vi "NET_speech.vi"(8 "error in (no error)":errorcluster, 10 "Голос":i32=1, 11 "textToSpeak":string="А всем привет!") -> (0 "error out":errorcluster, 2 "Голоса":T1(array[cluster]))   [LabVIEW 2017]
uses:
  System.Speech
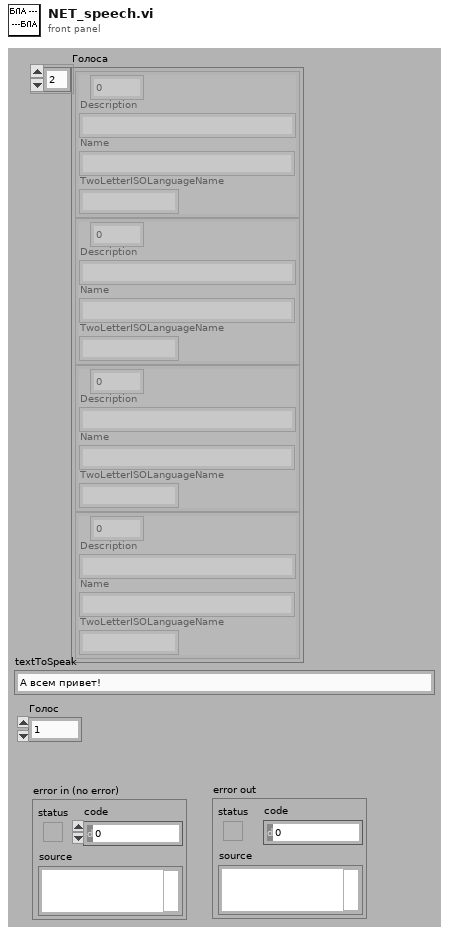
[diagram p1: front panel]
types:
  T1 = cluster{i32, "Description":string, "Name":string, "TwoLetterISOLanguageName":string}[]
  T2 = cluster{i32, "Description":string, "Name":string, "TwoLetterISOLanguageName":string}
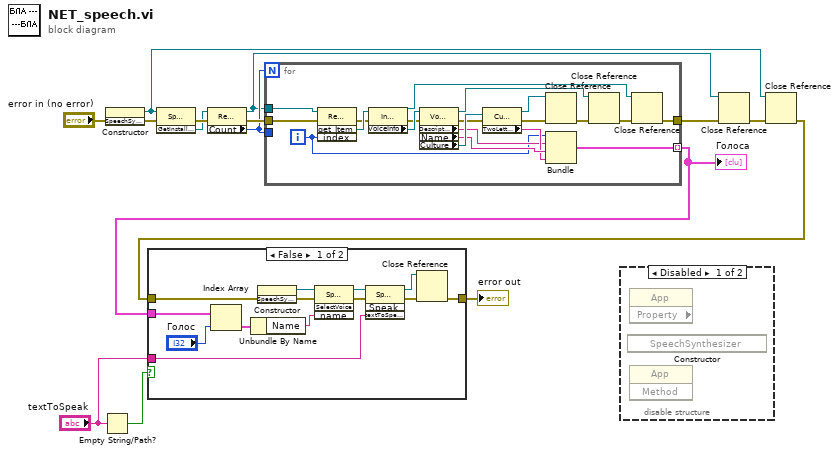
[diagram p0: block diagram]
diagram:
  n1 = Empty String/Path?(string/path="textToSpeak") -> (empty?=w5:bool)
  n2 = constructor class="SpeechSynthesizer"(error in="error in (no error)") -> (reference out=w7:refnum<k24>, error out=w15:errorcluster)  [unwired: 2 in, 1 out]
  n3 = invoke class="SpeechSynthesizer" method="GetInstalledVoices"(reference=w7, error in=w15) -> (error out=w14:errorcluster, "GetInstalledVoices"=w11:refnum<k24>)  [unwired: 1 in, 1 out]
  n4 = property class="ReadOnlyCollection`1[[System.Sp"(reference=w11, error in=w14) -> (reference out=w9:refnum<k24>, error out=w13:errorcluster, "Count"=w10:i32)
  n5 = for {
    N: w10 -> [_]
    tunnel: w9 -> [w35]
    tunnel: w10 -> [_]
    tunnel: [w28] -> w1 mode=indexing
    tunnel: w13 -> [w27]
    tunnel: [w17] -> w12
    i -> [w16]
    n6 = invoke class="ReadOnlyCollection`1[[System.Sp" method="get_Item"(reference=w35, error in=w27, "index"=w16) -> (error out=w26:errorcluster, "get_Item"=w34:refnum<k24>)  [unwired: 1 in, 2 out]
    n7 = property class="InstalledVoice"(reference=w34, error in=w26) -> (reference out=w18:refnum<k24>, error out=w25:errorcluster, "VoiceInfo"=w33:refnum<k24>)
    n8 = property class="VoiceInfo"(reference=w33, error in=w25) -> (reference out=w20:refnum<k24>, error out=w24:errorcluster, "Description"=w29:string, "Name"=w31:string, "Culture"=w32:refnum<k24>)
    n9 = property class="CultureInfo"(reference=w32, error in=w24) -> (reference out=w23:refnum<k24>, error out=w22:errorcluster, "TwoLetterISOLanguageName"=w30:string)
    n10 = Close Reference(reference=w23, error in (no error)=w22) -> (error out=w21:errorcluster)
    n11 = Bundle(w16, "Description"=w29, "Name"=w31, "TwoLetterISOLanguageName"=w30) -> (w28:T2)  [unwired: 1 out]
    n12 = Close Reference(reference=w20, error in (no error)=w21) -> (error out=w19:errorcluster)
    n13 = Close Reference(reference=w18, error in (no error)=w19) -> (error out=w17:errorcluster)
  }
  "Голоса" <- w1
  n14 = disable-structure shown="Disabled" {
    frame Disabled {
      n15 = constructor class="SpeechSynthesizer"() -> ()  [unwired: 3 in, 3 out]
      n16 = property class="App" props=[]() -> ()  [unwired: 2 in, 3 out]
      n17 = invoke class="App" method=#-1() -> ()  [unwired: 3 in, 3 out]
    }
    frame Enabled {
    }
  }
  n18 = Close Reference(reference=w9, error in (no error)=w12) -> (error out=w8:errorcluster)
  n19 = Close Reference(reference=w7, error in (no error)=w8) -> (error out=w4:errorcluster)
  n20 = case shown="False" w5 {
    tunnel: "textToSpeak" -> [w46 _]
    tunnel: w4 -> [w41 w49]
    tunnel: [w40 w49] -> w2
    tunnel: w1 -> [w37 _]
    frame False {
      n21 = Index Array(array=w37, index="Голос") -> (element=w39:T2)
      n22 = Unbundle By Name(w39) -> ("Name"=w36:string)
      n23 = constructor class="SpeechSynthesizer"(error in=w41) -> (reference out=w48:refnum<k24>, error out=w44:errorcluster)  [unwired: 2 in, 1 out]
      n24 = invoke class="SpeechSynthesizer" method="SelectVoice"(reference=w48, error in=w44, "name"=w36) -> (reference out=w47:refnum<k24>, error out=w43:errorcluster)  [unwired: 1 in, 2 out]
      n25 = invoke class="SpeechSynthesizer" method="Speak"(reference=w47, error in=w43, "textToSpeak"=w46) -> (reference out=w45:refnum<k24>, error out=w42:errorcluster)  [unwired: 1 in, 2 out]
      n26 = Close Reference(reference=w45, error in (no error)=w42) -> (error out=w40:errorcluster)
    }
    frame True {
    }
  }
  "error out" <- w2
